vi "DaqAnalog_Configuration.vi"(7 "Sampling Frequency":dbl=1000.0 format="%0.2f", 8 "error in":errorcluster, 9 "Number of Samples":i32=1000, 10 "Canales":tag[](array[tag]), 11 "DAQ Board Name":tag) -> (0 "error out":errorcluster, 3 "task out":refnum<k21>)   [LabVIEW 2020]
uses:
  <vilib>/DAQmx/create/channels.llb/DAQmx Create Channel (AI-Voltage-Basic).vi
  <vilib>/DAQmx/configure/timing.llb/DAQmx Timing (Sample Clock).vi
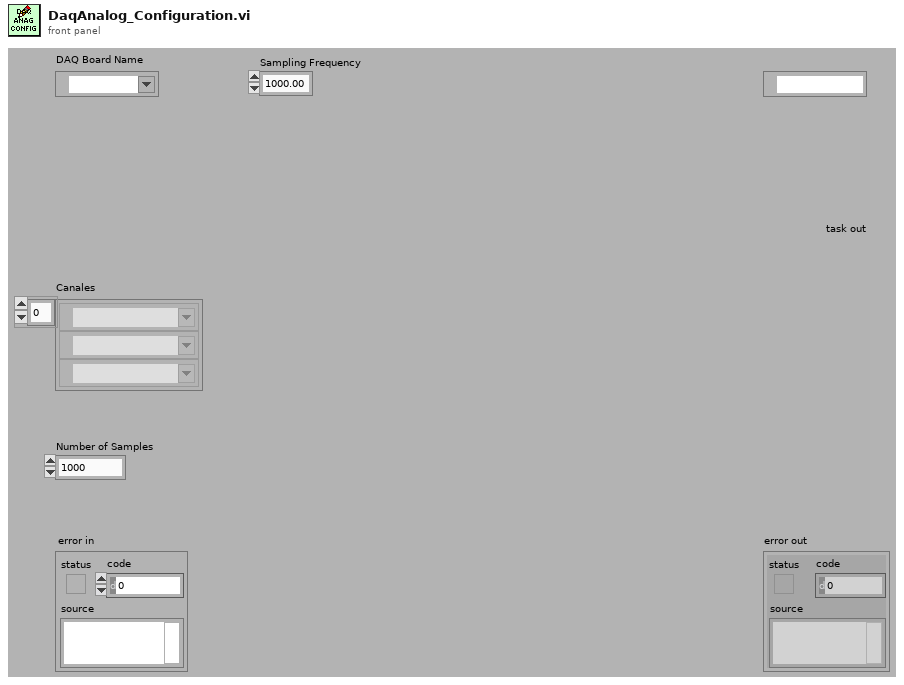
[diagram p1: front panel]
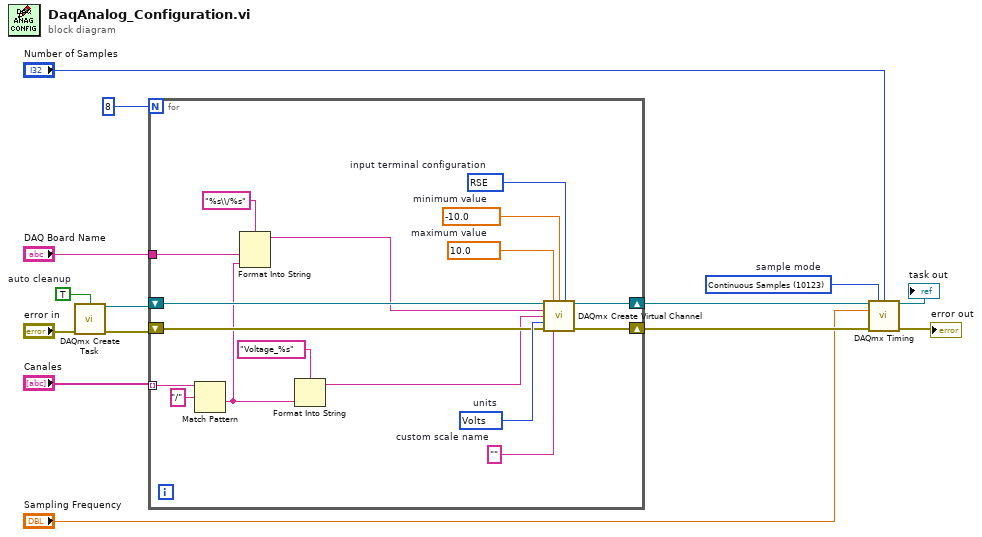
[diagram p0: block diagram]
diagram:
  w13 = 10123 items=["Finite Samples"=10178, "Continuous Samples"=10123, "Hardware Timed Single Point"=12522]  # sample mode
  w14 = TRUE  # auto cleanup
  n1 = call <vilib>:"DAQmx Create Task.vi"("auto cleanup"=w14, "error in"="error in") -> ("task out"=w11:refnum<k21>, "error out"=w10:errorcluster)  [unwired: 12 in]
  n2 = for {
    N: 8 -> [_]
    tunnel: "DAQ Board Name" -> [w24]
    tunnel: "Canales" -> [w22] mode=indexing
    shift-right: [w16] -> w8
    shift-left: w11 -> [w26]
    shift-right: [w15] -> w7
    shift-left: w10 -> [w25]
    w31 = 10083 items=["default"=-1, "RSE"=10083, "NRSE"=10078, "Differential"=10106, "Pseudodifferential"=12529]  # input terminal configuration
    w30 = 10348 items=["Volts"=10348, "From Custom Scale"=10065]  # units
    w29 = ""  # custom scale name
    w28 = -10.0  # minimum value
    w27 = 10.0  # maximum value
    n3 = Match Pattern(string=w22, regular expression="/") -> (after substring=w20:string)  [unwired: 1 in, 3 out]
    n4 = Format Into String(format string="%s\\/%s", w24, w20) -> (resulting string=w17:string)  [unwired: 2 in, 1 out]
    n5 = Format Into String(format string="Voltage_%s", w20) -> (resulting string=w18:string)  [unwired: 2 in, 1 out]
    n6 = call-poly <vilib>:"DAQmx Create Virtual Channel.vi"("task in"=w26, "maximum value"=w27, "minimum value"=w28, "input terminal configuration"=w31, "physical channels"=w17, "name to assign"=w18, "units"=w30, "error in"=w25, "custom scale name"=w29) -> ("task out"=w16:refnum<k21>, "error out"=w15:errorcluster)  [unwired: 5 in]
  }
  n7 = call-poly <vilib>:"DAQmx Timing.vi"("task/channels in"=w8, "sample mode"=w13, "samples per channel"="Number of Samples", "rate"="Sampling Frequency", "error in"=w7) -> ("task out"=→"task out":refnum<k21>, "error out"=→"error out":errorcluster)  [unwired: 9 in]
